vi "CoreCommand.vi"(8 "error in (no error)":errorcluster, 9 "Data":variant, 10 "Msg":T1, 11 "DAQ_Module in":refnum<class "DAQ_Module.lvclass">) -> (0 "error out":errorcluster, 3 "DAQ_Module out":refnum<class "DAQ_Module.lvclass">)   [LabVIEW 2025, in "DAQ_Module.lvlib" / "DAQ_Module.lvclass"]
uses:
  DAQ_Module.lvclass
  D:/Hardware/Module/Module/Module/Module.lvclass
  Msg.ctl
  Msg&Data.ctl
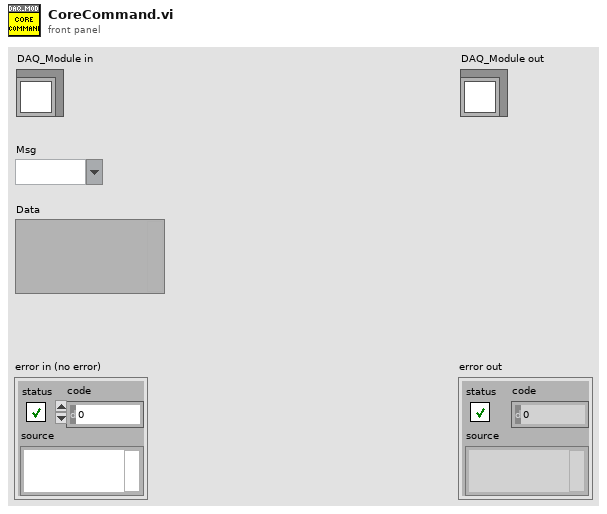
[diagram p1: front panel]
types:
  T1 = typedef "Msg.ctl" = string
  T2 = typedef "Msg&Data.ctl" = cluster{"Msg":T1, "Data":variant}
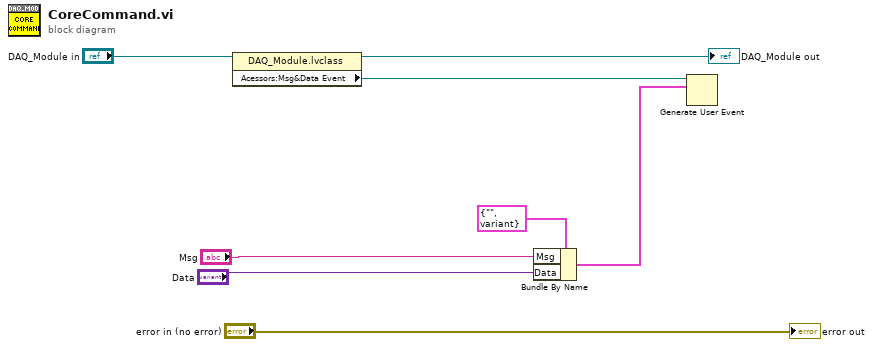
[diagram p0: block diagram]
diagram:
  n1 = property class="DAQ_Module.lvclass"(reference="DAQ_Module in") -> (reference out=→"DAQ_Module out":refnum<class "DAQ_Module.lvclass">, "Acessors:Msg&Data Event"=w1:refnum<user-event>)  [unwired: 1 in, 1 out]
  n2 = Bundle By Name(cluster=T2 {"Msg"="", "Data"=variant} ("Msg&Data"), "Msg"="Msg", "Data"="Data") -> (w7:T2)
  n3 = Generate User Event(user event=w1, event data cluster=w7) -> ()  [unwired: 2 in, 2 out]
  "error out" <- "error in (no error)"
